vi "RVC Interpolation 3D Motion.vi"() -> ()   [LabVIEW 2017]
uses:
  <vilib>/Analysis/baseanly.llb/Dot Product.vi
  <vilib>/Analysis/baseanly.llb/Real Dot Product.vi
  <vilib>/robotics/Kinematics/RotateX.vi
  <vilib>/robotics/Kinematics/RotateY.vi
  <vilib>/robotics/Kinematics/RotateZ.vi
  <vilib>/Analysis/baseanly.llb/A x B.vi
  <vilib>/Analysis/baseanly.llb/Real A x B.vi
  <vilib>/robotics/Kinematics/Rotation Matrix to Angle Vector.vi
  <vilib>/robotics/Kinematics/NI_Kinematics.lvlib
panel:
  out "Quaternion":refnum<vi>(3d-picture)
  out "RPY":refnum<vi>(3d-picture)
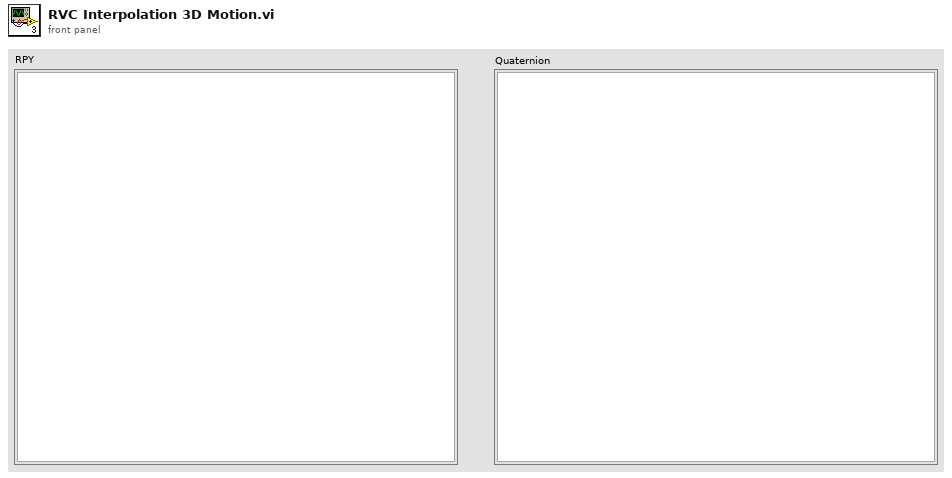
[diagram p1: front panel]
types:
  T1 = typedef "NI_Matrix.lvlib/RealMatrix.ctl" = dbl[][]
  T2 = typedef "NI_Kinematics.lvlib/Quaternion.ctl" = dbl[]
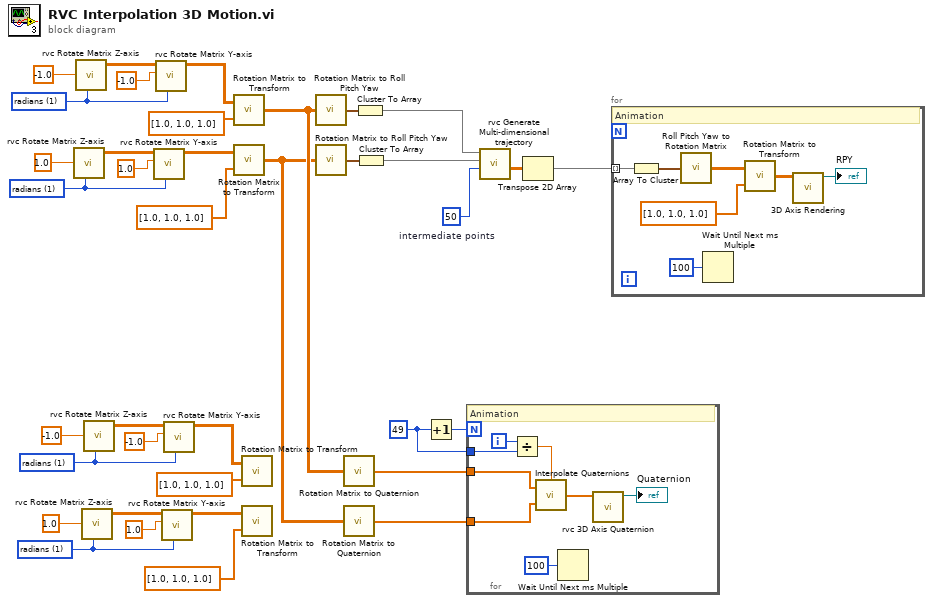
[diagram p0: block diagram]
diagram:
  w4 = 49
  w12 = u16 1 items=["degree", "radians"] ("angle unit")
  w13 = u16 1 items=["degree", "radians"] ("angle unit")
  w24 = u16 1 items=["degree", "radians"] ("angle unit")
  w25 = u16 1 items=["degree", "radians"] ("angle unit")
  w37 = 50  # intermediate points
  n1 = call "rvc Rotate Matrix Z-axis.vi"("angle unit"=w24, "angle"=1.0) -> ("rotation matrix"=w22:T1)  [unwired: 9 in]
  n2 = call "rvc Rotate Matrix Z-axis.vi"("angle unit"=w25, "angle"=-1.0) -> ("rotation matrix"=w28:T1)  [unwired: 9 in]
  n3 = call "rvc Rotate Matrix Z-axis.vi"("angle unit"=w12, "angle"=1.0) -> ("rotation matrix"=w10:T1)  [unwired: 9 in]
  n4 = call "rvc Rotate Matrix Z-axis.vi"("angle unit"=w13, "angle"=-1.0) -> ("rotation matrix"=w16:T1)  [unwired: 9 in]
  n5 = call "rvc Rotate Matrix Y-axis.vi"("angle unit"=w24, "angle"=1.0, "rotation matrix in"=w22) -> ("rotation matrix"=w20:T1)  [unwired: 8 in]
  n6 = call "rvc Rotate Matrix Y-axis.vi"("angle unit"=w25, "angle"=-1.0, "rotation matrix in"=w28) -> ("rotation matrix"=w26:T1)  [unwired: 8 in]
  n7 = call "rvc Rotate Matrix Y-axis.vi"("angle unit"=w12, "angle"=1.0, "rotation matrix in"=w10) -> ("rotation matrix"=w8:T1)  [unwired: 8 in]
  n8 = call "rvc Rotate Matrix Y-axis.vi"("angle unit"=w13, "angle"=-1.0, "rotation matrix in"=w16) -> ("rotation matrix"=w14:T1)  [unwired: 8 in]
  n9 = call <vilib>:"Rotation Matrix to Transform.vi"("translation vector"=dbl[] [1.0, 1.0, 1.0], "rotation matrix"=w26) -> ("transform"=w2:T1)
  n10 = call <vilib>:"Rotation Matrix to Transform.vi"("translation vector"=dbl[] [1.0, 1.0, 1.0], "rotation matrix"=w20) -> ("transform"=w1:T1)
  n11 = call <vilib>:"Rotation Matrix to Transform.vi"("translation vector"=dbl[] [1.0, 1.0, 1.0], "rotation matrix"=w14) -> ()  [unwired: 1 out]
  n12 = call <vilib>:"Rotation Matrix to Transform.vi"("translation vector"=dbl[] [1.0, 1.0, 1.0], "rotation matrix"=w8) -> ()  [unwired: 1 out]
  n13 = call <vilib>:"Rotation Matrix to Roll Pitch Yaw.vi"("rotation matrix"=w2) -> ("angles"=w33:cluster{"roll":dbl, "pitch":dbl, "yaw":dbl})
  n14 = call <vilib>:"Rotation Matrix to Roll Pitch Yaw.vi"("rotation matrix"=w1) -> ("angles"=w35:cluster{"roll":dbl, "pitch":dbl, "yaw":dbl})
  n15 = call <vilib>:"Rotation Matrix to Quaternion.vi"("rotation matrix"=w2) -> ("quaternion"=w6:T2)
  n16 = call <vilib>:"Rotation Matrix to Quaternion.vi"("rotation matrix"=w1) -> ("quaternion"=w5:T2)
  n17 = Cluster To Array(cluster=w33) -> (array=w32:dbl[])
  n18 = Cluster To Array(cluster=w35) -> (array=w34:dbl[])
  n19 = Increment(x=w4) -> (x+1=w3:i32)
  n20 = for {
    N: w3 -> [_]
    tunnel: w6 -> [w44]
    tunnel: w5 -> [w43]
    tunnel: w4 -> [w38]
    i -> [w42]
    # "Animation"
    n21 = Divide(x=w42, y=w38) -> (x/y=w39:dbl)
    n22 = call <vilib>:"Interpolate Quaternions.vi"("ratio"=w39, "quaternion 2"=w43, "quaternion 1"=w44) -> ("interpolated quaternion"=w41:T2)
    n23 = Wait Until Next ms Multiple(millisecond multiple=u32 100) -> ()  [unwired: 1 out]
    n24 = call "rvc 3D Axis Quaternion.vi"("quaternion"=w41) -> ("SceneNode out"=→"Quaternion":refnum<vi>)  [unwired: 10 in]
  }
  n25 = call "rvc Generate Multi-dimensional trajectory.vi"("number of timesteps"=w37, "final position array"=w34, "initial position array"=w32) -> ("multi-segment trajectories"=w36:dbl[][])  [unwired: 5 in, 3 out]
  n26 = Transpose 2D Array(2D array=w36) -> (transposed array=w31:dbl[][])
  n27 = for {
    tunnel: w31 -> [w51] mode=indexing
    # "Animation"
    n28 = Array To Cluster(array=w51) -> (cluster=w50:cluster{"[0]":dbl, "[1]":dbl, "[2]":dbl})
    n29 = call <vilib>:"Roll Pitch Yaw to Rotation Matrix.vi"("angles"=w50) -> ("rotation matrix"=w49:T1)
    n30 = Wait Until Next ms Multiple(millisecond multiple=u32 100) -> ()  [unwired: 1 out]
    n31 = call <vilib>:"Rotation Matrix to Transform.vi"("translation vector"=dbl[] [1.0, 1.0, 1.0], "rotation matrix"=w49) -> ("transform"=w48:T1)
    n32 = call "3D Axis Rendering.vi"("rotation matrix"=w48) -> ("SceneNode out"=→"RPY":refnum<vi>)  [unwired: 10 in]
  }
